vi "GET_send_AllServoData_toClient.vi"(3 "LabVIEW Web Service Request":refnum<class "Web Request.lvclass">) -> (0 "esp32Connected":bool, 1 "status":cluster{"mode":string, "position":dbl})   [LabVIEW 2024]
uses:
  <vilib>/wsapi/Web Request.lvclass
  DataTypes/OperationTypeForFunctionalGlobalVariable.ctl
  DataTypes/ServoStatus.ctl
  DataTypes/AllServoData.ctl
panel:
  out "?":cluster{"status":T1, "esp32Connected":bool} {"status"."position" min=0 max=180 step=1}
  # "Use the Web Service Request input terminal to call the VIs on the Web Services palette. Do not remove it from the connector pane unless you don't need access to the palette."
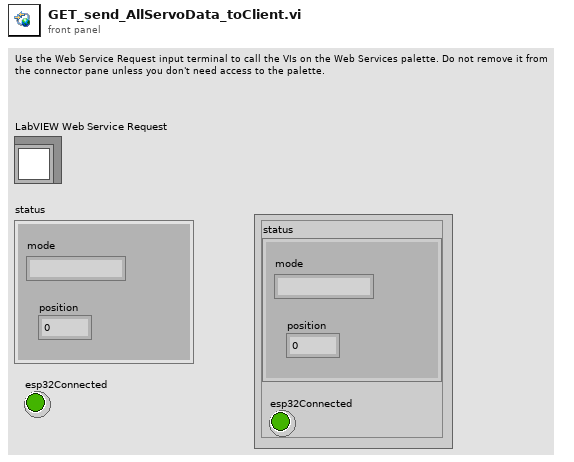
[diagram p1: front panel]
types:
  T1 = typedef "ServoStatus.ctl" = cluster{"mode":string, "position":i16}
  T2 = typedef "AllServoData.ctl" = cluster{"status":T1, "esp32Connected":bool}
  T3 = typedef "OperationTypeForFunctionalGlobalVariable.ctl" = enum16{"GET", "SET"}
  T4 = typedef "ServoConnectionStatus.ctl" = cluster{"esp32Connected":bool}
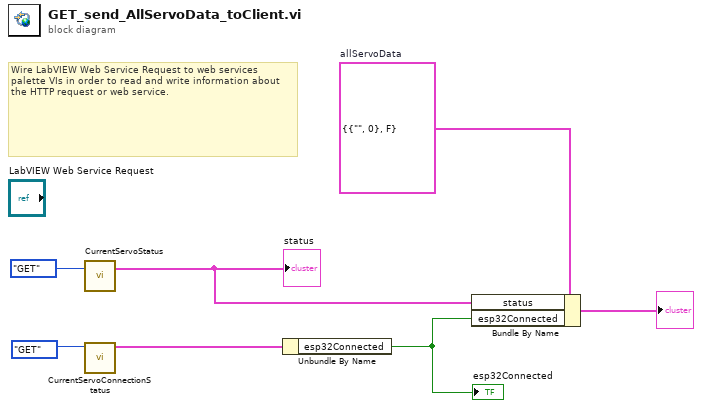
[diagram p0: block diagram]
diagram:
  w1 = T2 {"status"={"mode"="", "position"=0}, "esp32Connected"=FALSE}  # allServoData
  # "Wire LabVIEW Web Service Request to web services palette VIs in order to read and write information about the HTTP request or web service."
  n1 = call "CurrentServoStatus.vi"("Operation"=OperationTypeForFunctionalGlobalVariable."GET") -> ("Current Servo Status"=w4:T1)  [unwired: 2 in]
  "status" <- w4
  n2 = call "CurrentServoConnectionStatus.vi"("Operation"=OperationTypeForFunctionalGlobalVariable."GET") -> ("Current Servo Connection Status"=w5:T4)  [unwired: 10 in]
  n3 = Unbundle By Name(w5) -> ("esp32Connected"=w3:bool)
  "esp32Connected" <- w3
  n4 = Bundle By Name(cluster=w1, "status"=w4, "esp32Connected"=w3) -> (→"?":T2)
